vi "Run Action.vi"(7 "Logger":refnum<class "Logger.lvclass">, 8 "error in (no error)":errorcluster, 10 "Package":refnum<class "PackageAbstract.lvclass">, 11 "SyncAction in":refnum<class "SyncAction.lvclass">) -> (0 "error out":errorcluster, 2 "Problems":string[](array[string]), 3 "SyncAction out":refnum<class "SyncAction.lvclass">)   [LabVIEW 2020, in "GPackTools.lvlib" / "SyncAction.lvclass"]
uses:
  SyncAction.lvclass
  GPack/PackageAbstract/PackageAbstract.lvclass
  GPack/Logger/Logger.lvclass
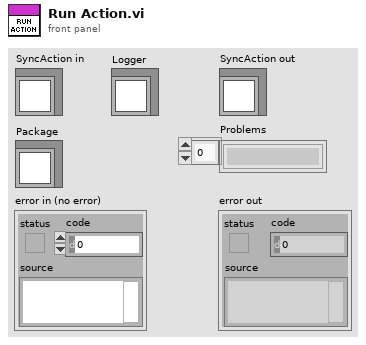
[diagram p1: front panel]
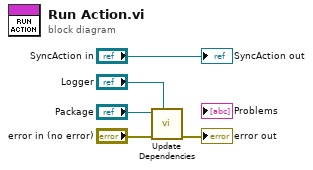
[diagram p0: block diagram]
diagram:
  n1 = call "Update Dependencies.vi"("Logger"="Logger", "error in (no error)"="error in (no error)", "PackageAbstract in"="Package") -> ("error out"=→"error out":errorcluster)  [unwired: 7 in, 1 out]
  "SyncAction out" <- "SyncAction in"
